vi "LV client.vi"() -> ()   [LabVIEW 2009]
uses:
  <vilib>/Utility/error.llb/DialogType.ctl
panel:
  out "Waveform Chart":dbl[][](graph)
  out "array":dbl[](array[numeric])
  out "remote address":string
  out "data out":string
  in  "Port":u16=9997
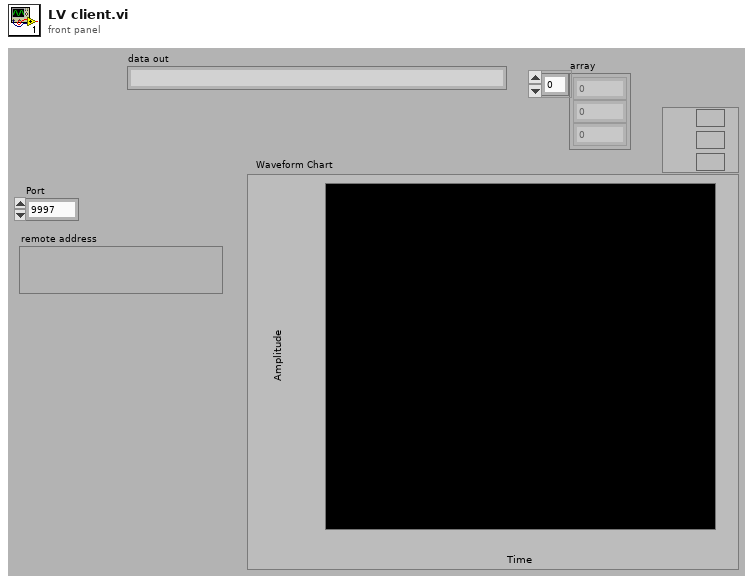
[diagram p1: front panel]
types:
  T1 = typedef "DialogType.ctl" = u16
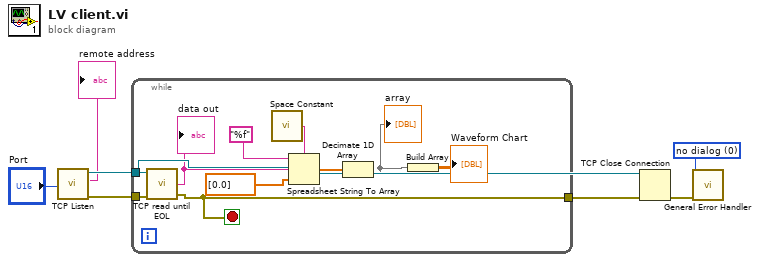
[diagram p0: block diagram]
diagram:
  w1 = T1 0 items=["no dialog", "OK message", "continue or stop message", "OK message + warnings", "continue/stop + warnings"] ("type of dialog (OK msg:1)")
  n1 = call <vilib>:"TCP Listen.vi"("port"="Port") -> ("error out"=w6:errorcluster, "remote address"=→"remote address":string, "connection ID"=w4:refnum<k5>)  [unwired: 7 in, 1 out]
  n2 = while {
    tunnel: w6 -> [w17]
    tunnel: [w15] -> w5
    tunnel: w4 -> [w16]
    stop <- w15 stop-if-true
    n3 = call "TCP read until EOL.vi"("error in (no error)"=w17, "connection ID"=w16) -> ("error out"=w15:errorcluster, "Final string"=w14:string)  [unwired: 2 in, 1 out]
    "data out" <- w14
    n4 = call <vilib>:"Space Constant.vi"() -> ("String"=w12:string)
    n5 = Spreadsheet String To Array(delimiter (Tab)=w12, format string="%f", spreadsheet string=w14, array type (2D Dbl)=dbl[] [0.0]) -> (array=w10:dbl[])
    n6 = Decimate 1D Array(w10) -> (w9:dbl[])  [unwired: 1 out]
    "array" <- w9
    n7 = Build Array(w9) -> (→"Waveform Chart":dbl[][])
  }
  n8 = TCP Close Connection(connection ID=w4, error in (no error)=w5) -> (error out=w2:errorcluster)  [unwired: 1 in, 1 out]
  n9 = call <vilib>:"General Error Handler.vi"("type of dialog (OK msg:1)"=w1, "error in (no error)"=w2) -> ()  [unwired: 9 in, 5 out]
